vi "Error Query.vi"(8 "error in (no error)":errorcluster, 11 "VISA resource name":refnum<visa-resource-name>) -> (0 "error out":errorcluster, 1 "Error Message":string, 2 "Error Code":i32[](array[numeric]), 3 "VISA resource name out":refnum<visa-resource-name>)   [LabVIEW 2020, in "MagnaDC.lvlib"]
doc: "Queries the instrument for any errors in the instrument's error queue. It will continue to read errors until all errors have been read from the instrument. Any errors will be returned in the <B>error out</B> control.\n\n<B>Note:</B>\nThis VI is called automatically by most driver VIs so it is not usually necessary to call this in an application."
uses:
  MagnaDC.lvlib
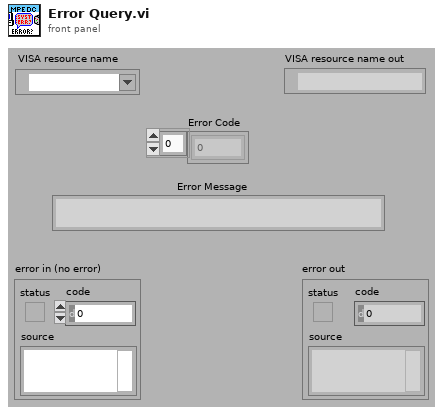
[diagram p1: front panel]
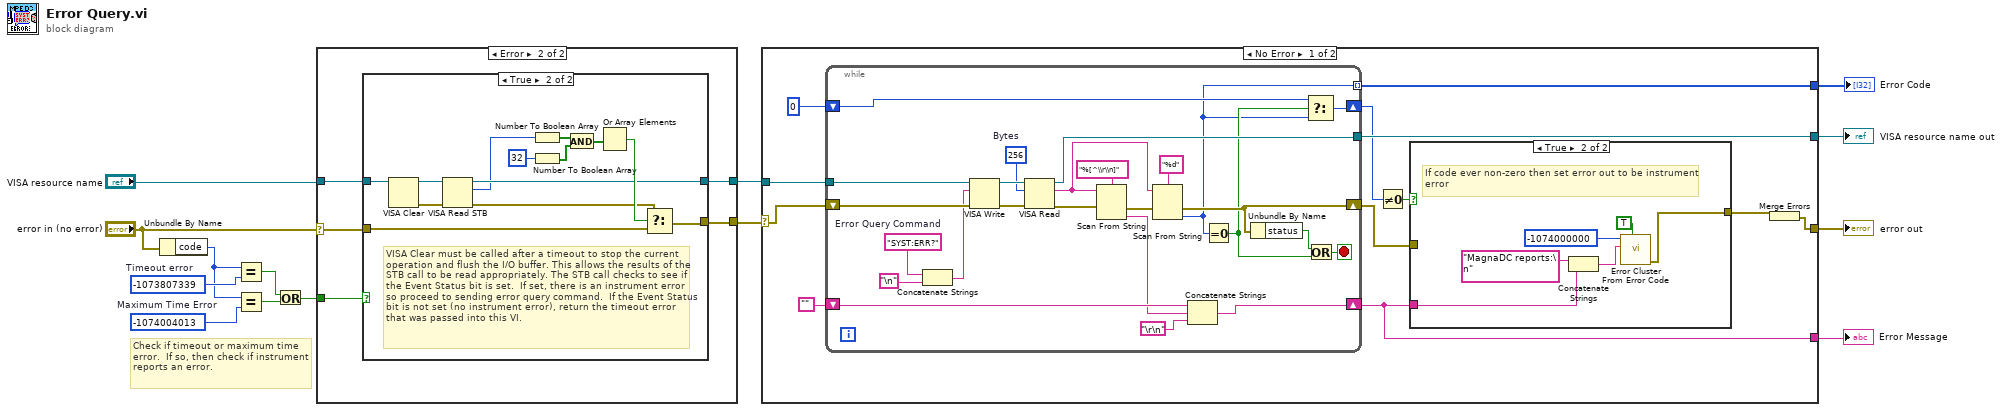
[diagram p0: block diagram]
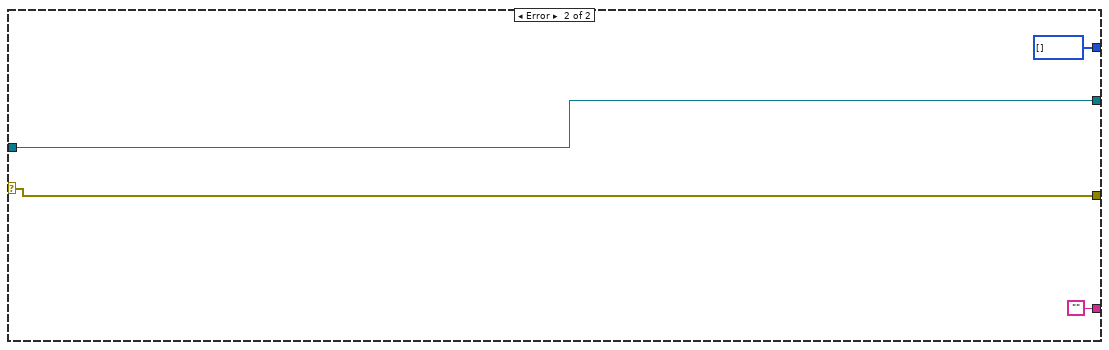
[diagram p5: hidden frame]
diagram:
  w5 = -1074004013  # Maximum Time Error
  w7 = -1073807339  # Timeout error
  # "Check if timeout or maximum time error.  If so, then check if instrument reports an error."
  n1 = Unbundle By Name("error in (no error)") -> ("code"=w6:i32)
  n2 = Equal?(x=w6, y=w7) -> (x = y?=w3:bool)
  n3 = Equal?(x=w6, y=w5) -> (x = y?=w4:bool)
  n4 = Or(x=w3, y=w4) -> (x .or. y?=w2:bool)
  n5 = case shown="Error" "error in (no error)" {
    selector: "error in (no error)" -> [w15 w19]
    tunnel: "VISA resource name" -> [w16 w21]
    tunnel: [w16 w20] -> w9
    tunnel: [w15 w18] -> w10
    tunnel: w2 -> [_ w17]
    frame No Error {
    }
    frame Error {
      n6 = case shown="True" w17 {
        tunnel: w21 -> [w23 w29]
        tunnel: [w23 w26] -> w20
        tunnel: w19 -> [w22 w32]
        tunnel: [w22 w31] -> w18
        frame False {
          # "Error code not a timeout, so best to pass on to user."
        }
        frame True {
          # "VISA Clear must be called after a timeout to stop the current operation and flush the I/O buffer. This allows the results of the  STB call to be read appropriately. The STB call checks to see if the Event Status bit is set.  If set, there is an instrument error so proceed to sending error query command.  If the Event Status bit is not set (no instrument error), return the timeout error that was passed into this VI."
          n7 = VISA Clear(VISA resource name=w29) -> (VISA resource name out=w28:refnum<visa-resource-name>, error out=w27:errorcluster)  [unwired: 1 in]
          n8 = VISA Read STB(8:w27, 11:w28) -> (0:w25:errorcluster, 2:w24:u16, 3:w26:refnum<visa-resource-name>)
          n9 = Number To Boolean Array(number=w24) -> (Boolean array=w33:bool[])
          n10 = Number To Boolean Array(number=32) -> (Boolean array=w35:bool[])
          n11 = And(x=w33, y=w35) -> (x .and. y?=w34:bool[])
          n12 = Or Array Elements(Boolean array=w34) -> (logical OR=w30:bool)
          n13 = Select(t=w25, s=w30, f=w32) -> (s? t:f=w31:errorcluster)
        }
      }
    }
  }
  n14 = case shown="No Error" w10 {
    selector: w10 -> [w37 w81]
    tunnel: [w48 w84] -> w14
    tunnel: w9 -> [w47 w84]
    tunnel: [w45 w81] -> w13
    tunnel: [w40 ""] -> w12
    tunnel: [w39 i32[] []] -> w11
    frame No Error {
      n15 = while {
        tunnel: [w80] -> w48
        tunnel: w47 -> [w79]
        shift-right: [w68] -> w40
        shift-left: "" -> [w71]
        shift-right: [w66] -> w41
        shift-left: 0 -> [w67]
        shift-right: [w64] -> w38
        shift-left: w37 -> [w65]
        tunnel: [w59] -> w39 mode=indexing
        stop <- w74 stop-if-true
        w77 = u32 256  # Bytes
        w57 = "SYST:ERR?"  # Error Query Command
        n16 = Concatenate Strings(w57, "\n") -> (w56:string)
        n17 = VISA Write(VISA resource name=w79, write buffer=w56, error in (no error)=w65) -> (VISA resource name out=w78:refnum<visa-resource-name>, error out=w76:errorcluster)  [unwired: 1 out]
        n18 = VISA Read(VISA resource name=w78, byte count=w77, error in (no error)=w76) -> (VISA resource name out=w80:refnum<visa-resource-name>, read buffer=w72:string, error out=w63:errorcluster)  [unwired: 1 out]
        n19 = Scan From String(format string="%[^\\r\\n]", input string=w72, error in=w63) -> (error out=w62:errorcluster, output 1=w69:string)  [unwired: 2 in, 2 out]
        n20 = Scan From String(format string="%d", input string=w72, error in=w62) -> (error out=w64:errorcluster, output 1=w59:i32)  [unwired: 2 in, 2 out]
        n21 = Concatenate Strings(w71, w69, "\r\n") -> (w68:string)
        n22 = Equal To 0?(x=w59) -> (x = 0?=w60:bool)
        n23 = Unbundle By Name(w64) -> ("status"=w61:bool)
        n24 = Select(t=w67, s=w60, f=w59) -> (s? t:f=w66:i32)
        n25 = Or(x=w61, y=w60) -> (x .or. y?=w74:bool)
      }
      n26 = Not Equal To 0?(x=w41) -> (x != 0?=w43:bool)
      n27 = case shown="True" w43 {
        tunnel: w40 -> [_ w54]
        tunnel: [w49 w50] -> w42
        tunnel: w38 -> [w49 _]
        frame False {
        }
        frame True {
          # "If code ever non-zero then set error out to be instrument error"
          n28 = Concatenate Strings("MagnaDC reports:\n" ("Source"), w54) -> (w51:string)
          n29 = call <vilib>:"Error Cluster From Error Code.vi"("show call chain? (False)"=TRUE, "error message (\"\")"=w51, "error code (0)"=-1074000000 ("Code")) -> ("error out"=w50:errorcluster)  [unwired: 6 in]
        }
      }
      n30 = Merge Errors(w42) -> (w45:errorcluster)
    }
    frame Error {
    }
  }
  "VISA resource name out" <- w14
  "error out" <- w13
  "Error Message" <- w12
  "Error Code" <- w11
